vi "Entry Console - Generate Wash Enclosure.vi"(8 "error in (no error)":errorcluster, 10 "Wash Step Selection buttons":T2, 11 "View Model":T3) -> (0 "error out":errorcluster, 2 "Wash Enclosure":T1[](array[typedef]), 3 "View Model":T3)   [LabVIEW 2017]
doc: "Transform Wash Step Selection buttons into array of wash steps"
uses:
  Model/Controls/View Model.ctl
  Model/Controls/Shared Model.ctl
  Error Handler/Controls/Error Model.ctl
  Error Handler/Controls/Error Message.ctl
  Error Handler/Controls/Error Type.ctl
  Configuration/Controls/Config Model.ctl
  Configuration/Controls/Config DB Message.ctl
  Configuration/Controls/Config DB Command.ctl
  Configuration/Controls/Config DB Overhead.ctl
  Configuration/Controls/Config DB Record.ctl
  Controller/Controls/Controller Model.ctl
  Vehicle Position Simulation/Controls/Vehicle - Position.ctl
  Controller/Controls/Controller Overhead.ctl
  Controller/Controls/Controller Wash Step.ctl
  Controls/Entry Console - Wash Step Select.ctl
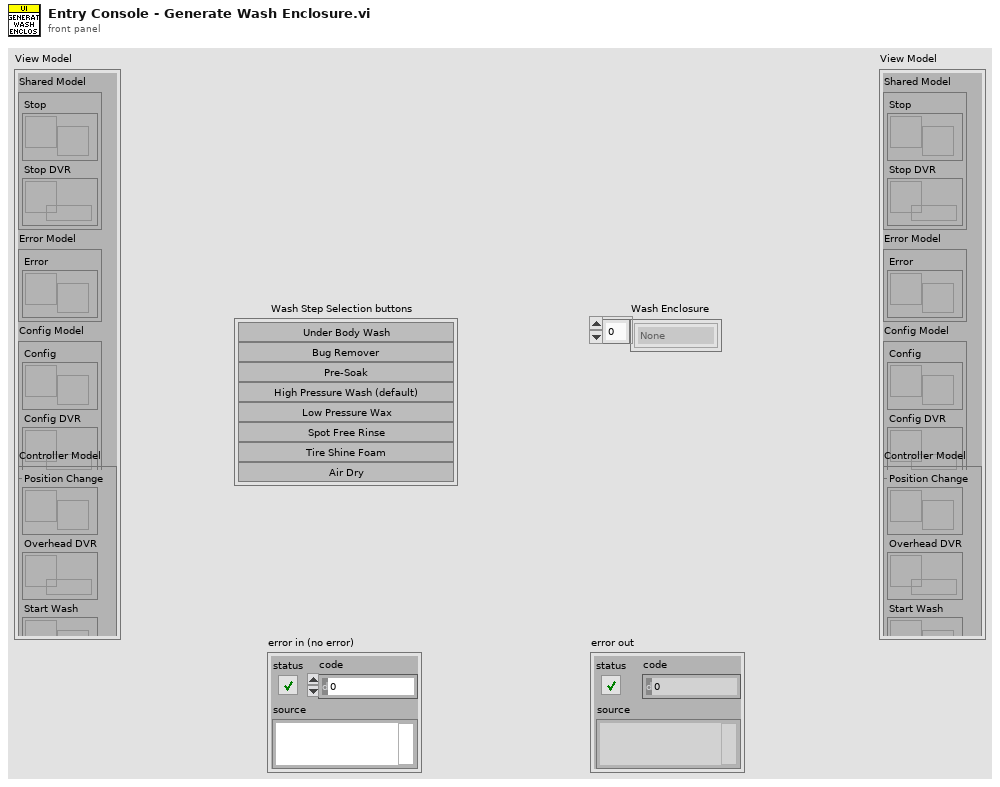
[diagram p1: front panel]
types:
  T1 = typedef "Controller Wash Step.ctl" = enum16{"None", "Under Body Wash", "Bug Remover", "Pre-Soak", "High Pressure Wash", "Low Pressure Wax", "Spot Free Rinse", "Tire Shine Foam", "Air Dry"}
  T2 = typedef "Entry Console - Wash Step Select.ctl" = cluster{"Under Body Wash":bool, "Bug Remover":bool, "Pre-Soak":bool, "High Pressure Wash":bool, "Low Pressure Wax":bool, "Spot Free Rinse":bool, "Tire Shine Foam":bool, "Air Dry":bool}
  T3 = typedef "View Model.ctl" = cluster{"Shared Model":T4, "Error Model":T5, "Config Model":T6, "Controller Model":T7}
  T4 = typedef "Shared Model.ctl" = cluster{"Stop":refnum<user-event>, "Stop DVR":refnum<data-value>}
  T5 = typedef "Error Model.ctl" = cluster{"Error":refnum<user-event>}
  T6 = typedef "Config Model.ctl" = cluster{"Config":refnum<user-event>, "Config DVR":refnum<data-value>}
  T7 = typedef "Controller Model.ctl" = cluster{"Position Change":refnum<user-event>, "Overhead DVR":refnum<data-value>, "Start Wash":refnum<user-event>}
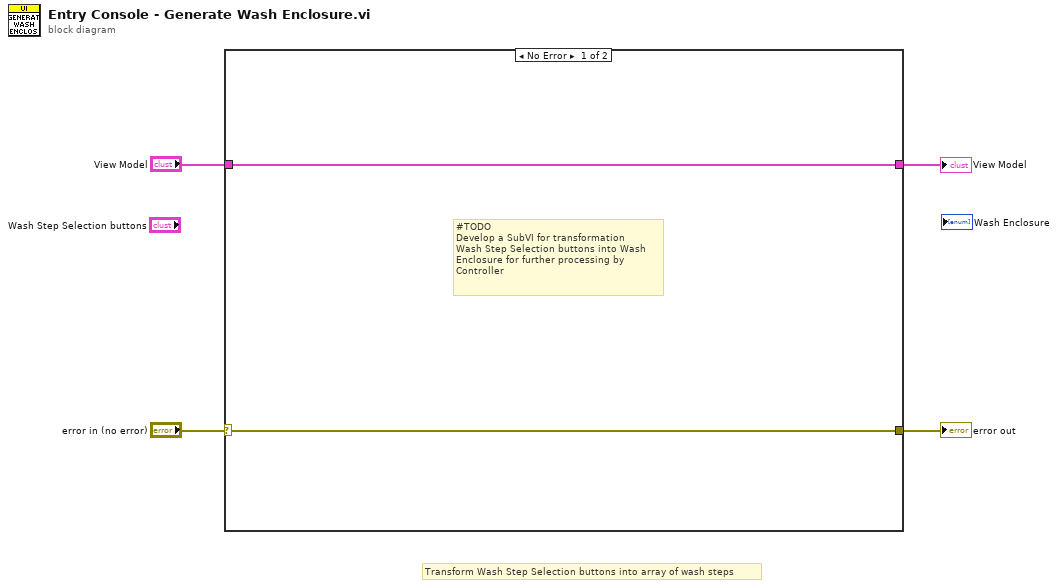
[diagram p0: block diagram]
diagram:
  # "Transform Wash Step Selection buttons into array of wash steps"
  n1 = case shown="No Error" "error in (no error)" {
    selector: "error in (no error)" -> [w6 w7]
    tunnel: "View Model" -> [w5 w8]
    tunnel: [w6 w7] -> w2
    tunnel: [w5 w8] -> w1
    frame No Error {
      # "#TODO\nDevelop a SubVI for transformation\nWash Step Selection buttons into Wash\nEnclosure for further processing by\nController"
    }
    frame Error {
    }
  }
  "View Model" <- w1
  "error out" <- w2
